vi "Thermal_Imager_GUI.vi"(11 "Snapshot":bool) -> ()   [LabVIEW 2015]
uses:
  <vilib>/userdefined/High Color/IMAQdx.ctl
  <vilib>/Instr/_visa.llb/VISA Configure Serial Port (Instr).vi
  <vilib>/vision/driver/NI_Vision_Acquisition_Software.lvlib
  <resource>/objmgr/imaqdx.rc
panel:
  out "Value":dbl
  in  "X Positions":string[][](table)=[["1", "1000"], ["2", "2000"], ["3", "4000"], ["4", "5000"]]
  out "Motor Response":string
  in  "flow control":u16
  in  "stop bits":u16=10
  in  "parity":u16
  in  "data bits":u16=8 min=5 max=8 step=1
  in  "COM port":refnum<visa-resource-name>="COM8"
  in  "baud rate":u32=57600
  in  "Interval (s)":u32=10
  out "error out 2":errorcluster
  in  "Runs":i32=3
  in  "Timelapse":bool
  in  "Save Directory":path=path "C:/Users/RoboLap/Desktop/test"
  out "Temp (°C)":dbl(slide)=25.5 scale=0.0..70.0
  out "Image":T1(plugin-control)
  in  "Stop":bool
  in  "Camera Session In":T2="cam0"
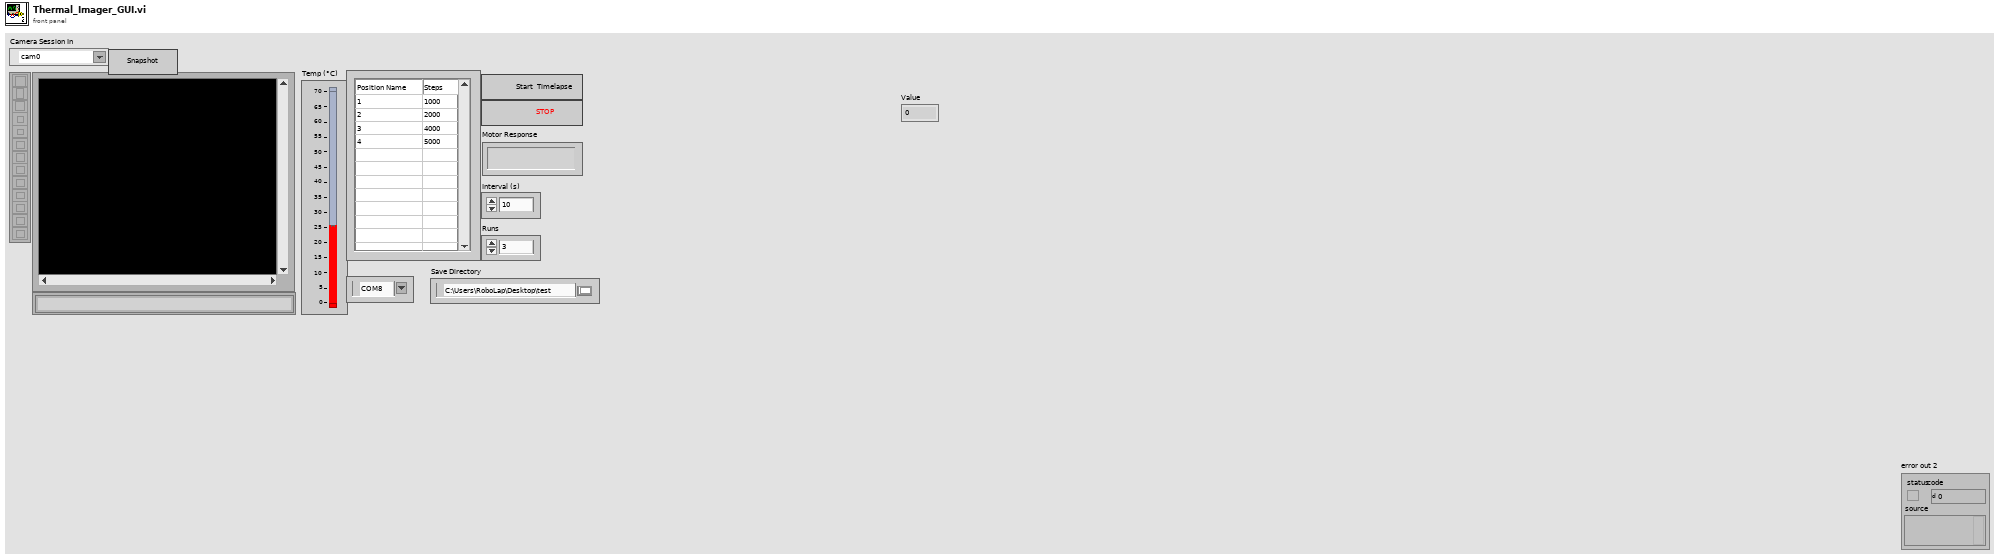
[diagram p1: front panel]
types:
  T1 = typedef "IMAQ Image.ctl" = refnum<image>
  T2 = typedef "IMAQdx.ctl" = refnum<k21>
  T3 = typedef "Image Type" = u32
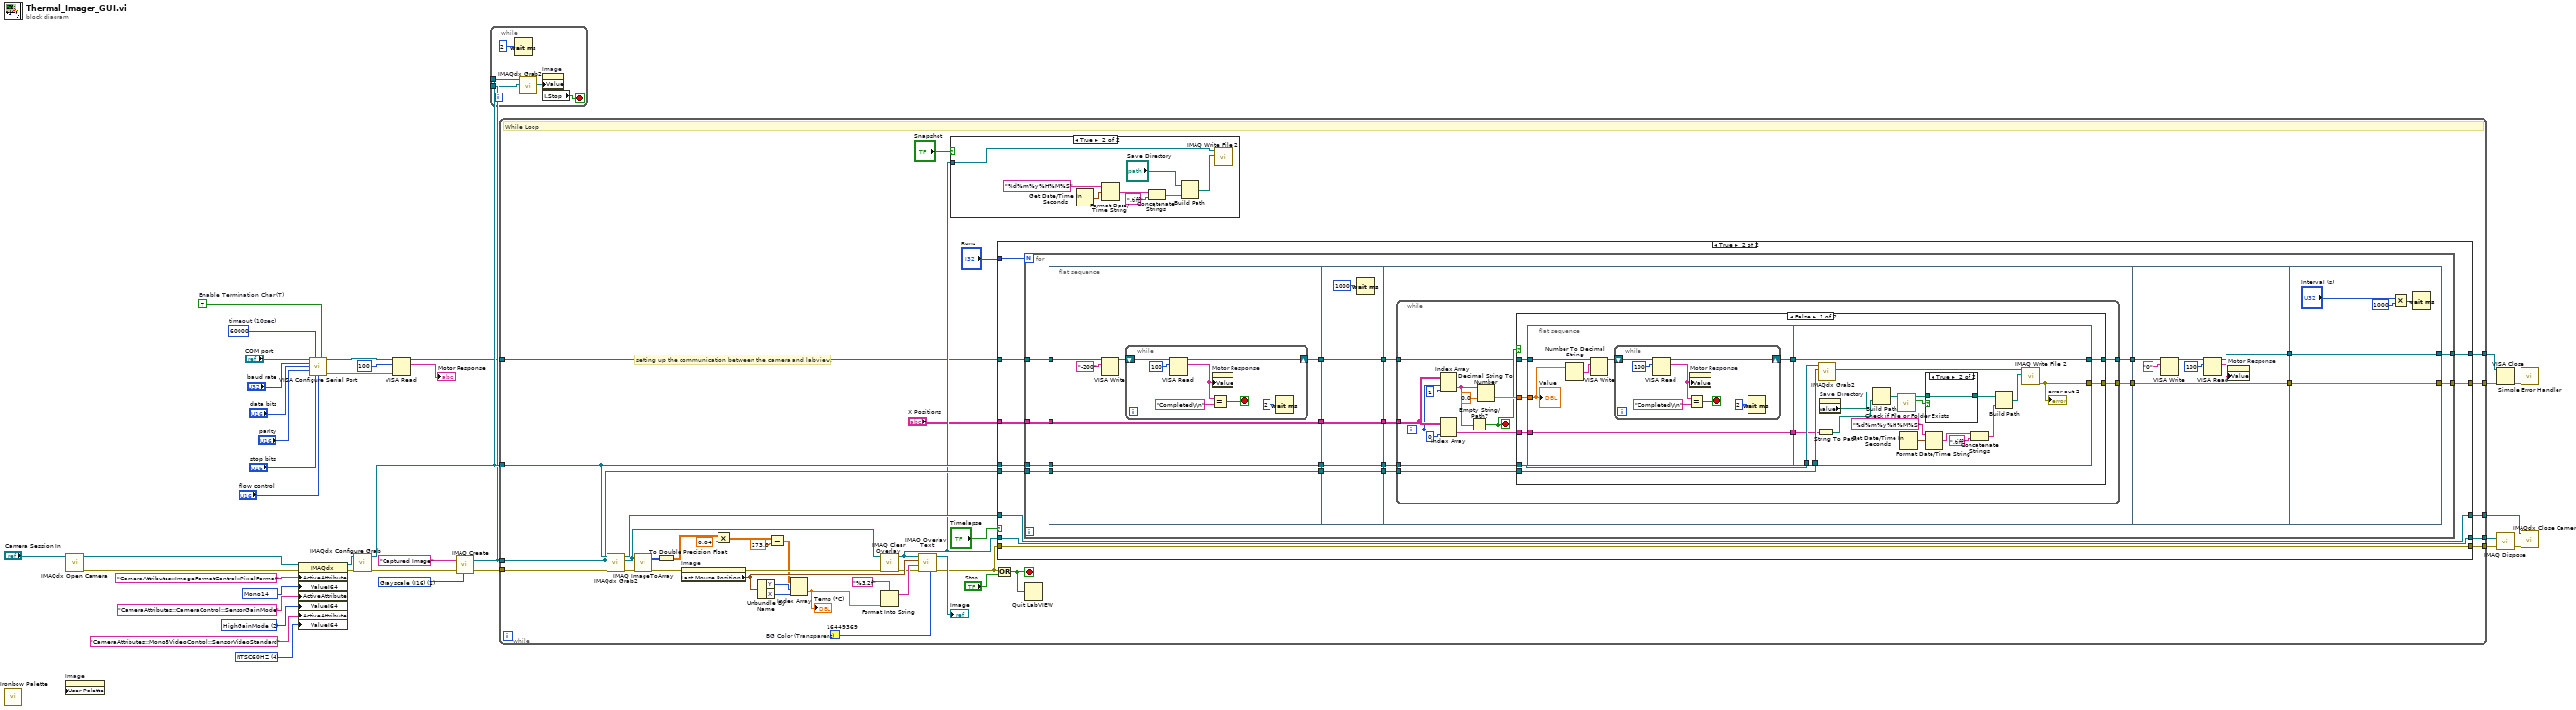
[diagram p0: block diagram]
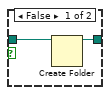
[diagram p3: hidden frame]
diagram:
  w13 = TRUE  # Enable Termination Char (T)
  w14 = u32 60000  # timeout (10sec)
  w30 = i64 4 items=["NTSC30HZ"=0, "PAL25Hz"=1, "NTSC60HZ"=4, "PAL50HZ"=5] ("IRFrameRate")
  w31 = i64 2 items=["LowGainMode"=1, "HighGainMode"=2] ("IRFormat")
  w32 = i64 17825829 items=["Mono 8"=17301505, "Mono14"=17825829, "Mono16"=17825799] ("Ring")
  w34 = T3 1 items=["Grayscale (U8)", "Grayscale (I16)", "Grayscale (SGL)", "Complex (CSG)", "RGB (U32)", "HSL (U32)", "RGB (U64)", "Grayscale (U16)"] ("Image Type")
  n1 = call "Ironbow Palette.vi"() -> ("Color Palette"=w1:cluster{"Red":u8, "Green":u8, "Blue":u8}[])  [unwired: 11 in]
  n2 = property on="Image" class="ImageControl"("User Palette"=w1) -> ()  [unwired: 2 in, 2 out]
  n3 = call <vilib>:"IMAQdx Open Camera.vi"("Session In"="Camera Session In") -> ("error out"=w37:errorcluster, "Session Out"=w33:T2)  [unwired: 9 in]
  n4 = property class="IMAQdx"(reference=w33, error in=w37, "ActiveAttribute"="CameraAttributes::ImageFormatControl::PixelFormat", "ValueI64"=w32, "ActiveAttribute"="CameraAttributes::CameraControl::SensorGainMode", "ValueI64"=w31, "ActiveAttribute"="CameraAttributes::Mono8VideoControl::SensorVideoStandard", "ValueI64"=w30) -> (reference out=w36:T2, error out=w29:errorcluster)
  n5 = call-poly "VISA Configure Serial Port"("VISA resource name"="COM port", "timeout (10sec)"=w14, "Enable Termination\nChar (T)"=w13, "baud rate (9600)"="baud rate", "data bits (8)"="data bits", "parity (0:none)"="parity", "stop bits (10: 1 bit)"="stop bits", "flow control (0:none)"="flow control") -> ("VISA resource name out"=w9:refnum<visa-resource-name>, "error out"=w8:errorcluster)  [unwired: 6 in]
  n6 = call <vilib>:"IMAQdx Configure Grab.vi"("error in"=w29, "Session In"=w36) -> ("error out"=w28:errorcluster, "Session Out"=w19:T2)  [unwired: 8 in]
  n7 = VISA Read(VISA resource name=w9, byte count=u32 100, error in (no error)=w8) -> (VISA resource name out=w2:refnum<visa-resource-name>, read buffer=→"Motor Response":string)  [unwired: 2 out]
  n8 = call "IMAQ Create"("Image Name"="Captured Image", "Image Type"=w34, "error in (no error)"=w28) -> ("New Image"=w18:T1, "error out"=w27:errorcluster)  [unwired: 2 in]
  n9 = while {
    tunnel: w19 -> [w42]
    tunnel: w18 -> [w41]
    stop <- w40 stop-if-true
    n10 = Wait (ms)(milliseconds to wait=u32 2 ("millisecond timer value")) -> ()  [unwired: 1 out]
    n11 = call <vilib>:"IMAQdx Grab2.vi"("Image In"=w41, "Session In"=w42) -> ("Image Out"=w43:T1)  [unwired: 6 in, 3 out]
    n12 = property on="Image" class="ImageControl"("Value"=w43) -> ()  [unwired: 2 in, 2 out]
    n13 = local read "Stop"() -> (w40:bool)
  }
  n14 = while {
    tunnel: w27 -> [w78]
    tunnel: w19 -> [w57]
    tunnel: w18 -> [w56]
    tunnel: [w49] -> w26
    tunnel: [w53] -> w21
    tunnel: [w51] -> w20
    tunnel: w2 -> [w48]
    tunnel: [w47] -> w6
    tunnel: [w46] -> w5
    stop <- w45 stop-if-true
    w71 = u32 16449369  # BG Color (Transparent)
    # "setting up the communication between the camera and labview."
    # "While Loop"
    n15 = call <vilib>:"IMAQdx Grab2.vi"("error in"=w78, "Image In"=w56, "Session In"=w57) -> ("error out"=w79:errorcluster, "Image Out"=w62:T1, "Session Out"=w54:T2)  [unwired: 5 in, 1 out]
    n16 = call "IMAQ ImageToArray"("error in (no error)"=w79, "Image"=w62) -> ("error out"=w77:errorcluster, "Image Pixels (I16)"=w64:i16[][])  [unwired: 2 in, 3 out]
    n17 = To Double Precision Float(number=w64) -> (double precision float=w76:dbl[][])
    n18 = property on="Image" class="ImageControl"(error in=w77) -> (error out=w69:errorcluster, "Last Mouse Position"=w70:cluster{"X":i32, "Y":i32})  [unwired: 1 in, 1 out]
    n19 = Multiply(x=w76, y=0.04) -> (x*y=w65:dbl[][])
    n20 = Unbundle By Name(w70) -> ("Y"=w66:i32, "X"=w67:i32)
    n21 = Subtract(x=w65, y=273.0) -> (x-y=w61:dbl[][])
    n22 = Index Array(array=w61, index (row)=w66, index (col)=w67) -> (element=w74:dbl)
    "Temp (°C)" <- w74
    n23 = call "IMAQ Clear Overlay"("error in (no error)"=w69, "Image"=w62) -> ("error out"=w68:errorcluster, "Image Out"=w52:T1)  [unwired: 8 in]
    n24 = Format Into String(format string="%3.2f", w74) -> (resulting string=w72:string)  [unwired: 2 in, 1 out]
    n25 = call "IMAQ Overlay Text"("BG Color (Transparent)"=w71, "error in (no error)"=w68, "String"=w72, "Origin"=w70, "Image"=w52) -> ("error out"=w50:errorcluster, "Image Out"=→"Image":T1)  [unwired: 5 in]
    n26 = case shown="True" "Snapshot" {
      tunnel: w52 -> [_ w207]
      frame False {
      }
      frame True {
        n27 = Get Date/Time In Seconds() -> (seconds since 1Jan1904=w214:timestamp)
        n28 = Format Date/Time String(time format string (%c)="%d%m%y%H%M%S", seconds (now)=w214) -> (date/time string=w208:string)  [unwired: 1 in]
        n29 = Concatenate Strings(w208, ".tiff" ("string")) -> (w211:string)
        n30 = Build Path(base path="Save Directory", name or relative path=w211) -> (appended path=w209:path)
        n31 = call-poly "IMAQ Write File 2"("File Path"=w209, "Image"=w207) -> ()  [unwired: 8 in, 2 out]
      }
    }
    n32 = Or(x=w50, y="Stop") -> (x .or. y?=w45:bool)
    n33 = case shown="True" "Timelapse" {
      tunnel: "Runs" -> [_ w93]
      tunnel: w57 -> [_ w88]
      tunnel: w56 -> [_ w89]
      tunnel: w54 -> [w83 w92]
      tunnel: [w83 w92] -> w53
      tunnel: w52 -> [w82 w91]
      tunnel: [w82 w91] -> w51
      tunnel: w50 -> [w81 w90]
      tunnel: [w81 w90] -> w49
      tunnel: w48 -> [_ w87]
      tunnel: [_ w86] -> w47
      tunnel: [_ w85] -> w46
      tunnel: "X Positions" -> [_ w84]
      frame False {
      }
      frame True {
        n34 = for {
          N: w93 -> [_]
          tunnel: w88 -> [w108]
          tunnel: w89 -> [w111]
          tunnel: w87 -> [w107]
          tunnel: [w110] -> w86
          tunnel: [w109] -> w85
          tunnel: w84 -> [w106]
          n35 = flat-sequence {
            tunnel: w111 -> [w117]
            tunnel: w108 -> [w118]
            tunnel: [w118] -> w97
            tunnel: [w117] -> w99
            tunnel: [w113] -> w101
            tunnel: w107 -> [w115]
            tunnel: [w112] -> w95
            tunnel: w106 -> [w112]
            tunnel: w101 -> [w130]
            tunnel: [w130] -> w100
            tunnel: w99 -> [w129]
            tunnel: [w129] -> w98
            tunnel: w97 -> [w128]
            tunnel: [w128] -> w96
            tunnel: w95 -> [w127]
            tunnel: [w127] -> w94
            tunnel: [w131] -> w105
            tunnel: w100 -> [w135]
            tunnel: w98 -> [w133]
            tunnel: w96 -> [w134]
            tunnel: w94 -> [w136]
            tunnel: [w132] -> w103
            tunnel: w105 -> [w201]
            tunnel: [w201] -> w104
            tunnel: w103 -> [w195]
            tunnel: [w196] -> w102
            tunnel: [w203] -> w110
            tunnel: [w202] -> w109
            tunnel: w104 -> [w202]
            tunnel: w102 -> [w203]
            frame #0 {
              n36 = VISA Write(VISA resource name=w115, write buffer="-200") -> (VISA resource name out=w114:refnum<visa-resource-name>)  [unwired: 1 in, 2 out]
              n37 = while {
                shift-right: [w124] -> w113
                shift-left: w114 -> [w125]
                stop <- w120 stop-if-true
                n38 = VISA Read(VISA resource name=w125, byte count=u32 100) -> (VISA resource name out=w124:refnum<visa-resource-name>, read buffer=w122:string)  [unwired: 1 in, 2 out]
                n39 = Equal?(x=w122, y="Completed\r\n") -> (x = y?=w120:bool)
                n40 = property on="Motor Response" class="Str"("Value"=w122) -> ()  [unwired: 2 in, 2 out]
                n41 = Wait (ms)(milliseconds to wait=u32 2) -> ()  [unwired: 1 out]
              }
            }
            frame #1 {
              n42 = Wait (ms)(milliseconds to wait=u32 1000 ("millisecond timer value")) -> ()  [unwired: 1 out]
            }
            frame #2 {
              n43 = while {
                tunnel: w136 -> [w146]
                tunnel: w135 -> [w142]
                tunnel: [w141] -> w132
                tunnel: w134 -> [w140]
                tunnel: w133 -> [w139]
                tunnel: [w138] -> w131
                i -> [w144]
                stop <- w143 stop-if-true
                n44 = Index Array(array=w146, index (row)=w144, index (col)=1 ("disabled index (col)")) -> (element=w149:string)
                n45 = Index Array(array=w146, index (row)=w144, index (col)=0 ("disabled index (col)")) -> (element=w137:string)
                n46 = Empty String/Path?(string/path=w149) -> (empty?=w143:bool)
                n47 = Decimal String To Number(string=w149, default (0L)=0.0) -> (number=w147:dbl)  [unwired: 1 in, 1 out]
                n48 = case shown="False" w143 {
                  tunnel: w147 -> [w159 _]
                  tunnel: w142 -> [w158 w194]
                  tunnel: [w157 w194] -> w141
                  tunnel: w140 -> [w155 _]
                  tunnel: w139 -> [w154 _]
                  tunnel: [w153 _] -> w138
                  tunnel: w137 -> [w151 _]
                  frame False {
                    n49 = flat-sequence {
                      tunnel: w158 -> [w163]
                      tunnel: w159 -> [w165]
                      tunnel: [w162] -> w156
                      tunnel: [w160] -> w152
                      tunnel: w151 -> [w160]
                      tunnel: [w190] -> w153
                      tunnel: [w189] -> w157
                      tunnel: w152 -> [w173]
                      tunnel: w154 -> [w187]
                      tunnel: w155 -> [w188]
                      tunnel: w156 -> [w189]
                      frame #0 {
                        n50 = Number To Decimal String(number=w165) -> (decimal integer string=w161:string)  [unwired: 1 in]
                        n51 = VISA Write(VISA resource name=w163, write buffer=w161) -> (VISA resource name out=w164:refnum<visa-resource-name>)  [unwired: 1 in, 2 out]
                        n52 = while {
                          shift-right: [w170] -> w162
                          shift-left: w164 -> [w172]
                          stop <- w167 stop-if-true
                          n53 = VISA Read(VISA resource name=w172, byte count=u32 100) -> (VISA resource name out=w170:refnum<visa-resource-name>, read buffer=w169:string)  [unwired: 1 in, 2 out]
                          n54 = Equal?(x=w169, y="Completed\r\n") -> (x = y?=w167:bool)
                          n55 = property on="Motor Response" class="Str"("Value"=w169) -> ()  [unwired: 2 in, 2 out]
                          n56 = Wait (ms)(milliseconds to wait=u32 2 ("millisecond timer value")) -> ()  [unwired: 1 out]
                        }
                        "Value" <- w165
                      }
                      frame #1 {
                        n57 = String To Path(string=w173) -> (path=w181:path)
                        n58 = call <vilib>:"IMAQdx Grab2.vi"("Image In"=w187, "Session In"=w188) -> ("Image Out"=w174:T1)  [unwired: 6 in, 3 out]
                        n59 = property on="Save Directory" class="Path"() -> ("Value"=w180:path)  [unwired: 2 in, 2 out]
                        n60 = Build Path(base path=w180, name or relative path=w181) -> (appended path=w183:path)
                        n61 = call <vilib>:"Check if File or Folder Exists.vi"("path"=w183) -> ("file or folder exists?"=w184:bool, "dup path"=w185:path)  [unwired: 8 in, 1 out]
                        n62 = Get Date/Time In Seconds() -> (seconds since 1Jan1904=w175:timestamp)
                        n63 = case shown="True" w184 {
                          tunnel: w185 -> [w192 w193]
                          tunnel: [w191 w193] -> w186
                          frame False {
                            n64 = Create Folder(path (use dialog)=w192) -> (created path=w191:path)  [unwired: 2 in, 2 out]
                          }
                          frame True {
                          }
                        }
                        n65 = Format Date/Time String(time format string (%c)="%d%m%y%H%M%S", seconds (now)=w175) -> (date/time string=w179:string)  [unwired: 1 in]
                        n66 = Concatenate Strings(w179, ".tiff" ("string")) -> (w182:string)
                        n67 = Build Path(base path=w186, name or relative path=w182) -> (appended path=w178:path)
                        n68 = call-poly "IMAQ Write File 2"("File Path"=w178, "Image"=w174) -> ("error out"=w190:errorcluster)  [unwired: 8 in, 1 out]
                        "error out 2" <- w190
                      }
                    }
                  }
                  frame True {
                  }
                }
              }
            }
            frame #3 {
              n69 = VISA Write(VISA resource name=w195, write buffer="0") -> (VISA resource name out=w198:refnum<visa-resource-name>)  [unwired: 1 in, 2 out]
              n70 = VISA Read(VISA resource name=w198, byte count=u32 100) -> (VISA resource name out=w196:refnum<visa-resource-name>, read buffer=w200:string)  [unwired: 1 in, 2 out]
              n71 = property on="Motor Response" class="Str"("Value"=w200) -> ()  [unwired: 2 in, 2 out]
            }
            frame #4 {
              n72 = Multiply(x="Interval (s)", y=u32 1000) -> (x*y=w205:u32)
              n73 = Wait (ms)(milliseconds to wait=w205) -> ()  [unwired: 1 out]
            }
          }
        }
      }
    }
    n74 = Quit LabVIEW(quit? (T)=w45) -> ()
  }
  n75 = VISA Close(VISA resource name=w6, error in (no error)=w5) -> (error out=w7:errorcluster)
  n76 = call "IMAQ Dispose"("Image"=w20, "error in (no error)"=w26) -> ("error out"=w25:errorcluster)  [unwired: 4 in]
  n77 = call <vilib>:"Simple Error Handler.vi"("error in (no error)"=w7) -> ()  [unwired: 4 in, 5 out]
  n78 = call <vilib>:"IMAQdx Close Camera.vi"("error in"=w25, "Session In"=w21) -> ()  [unwired: 9 in, 1 out]
